vi "loadTestsFromTestCases.vi"(7 "testSuiteStatusChangedRef":refnum<user-event>, 8 "error in (no error)":errorcluster, 10 "Tests":refnum<class>[](array[class]), 11 "TestLoader in":refnum<class "TestLoader.lvclass">) -> (0 "error out":errorcluster, 2 "TestSuite":refnum<class "TestSuite.lvclass">, 3 "TestLoader out":refnum<class "TestLoader.lvclass">)   [LabVIEW 2019, in "TestLoader.lvclass"]
uses:
  TestLoader.lvclass
  TestSuite/TestSuite.lvclass
  TestSuite/suiteStatusChanged--Cluster.ctl
  TestSuite/suiteStatus--enum.ctl
  TestCase/TestCase.lvclass
  <userlib>/_OpenG.lib/array/array.llb/Conditional Auto-Indexing Tunnel (LVObject)__ogtk.vi
  <userlib>/_OpenG.lib/array/array.llb/Conditional Auto-Indexing Tunnel (Variant)__ogtk.vi
  <userlib>/_OpenG.lib/array/array.llb/Filter 1D Array (String)__ogtk.vi
  <userlib>/_OpenG.lib/array/array.llb/Remove Duplicates from 1D Array (I32)__ogtk.vi
  <userlib>/_OpenG.lib/array/array.llb/Delete Elements from 1D Array (LVObject)__ogtk.vi
  Libraries/VITesterUtilities.lvlib
panel:
  # "JKI VI Tester for LabVIEW\nhttp://jkisoft.com/vi-tester\nCopyright (C) 2007-2009, JKI <info@jkisoft.com>\nALL RIGHTS RESERVED"
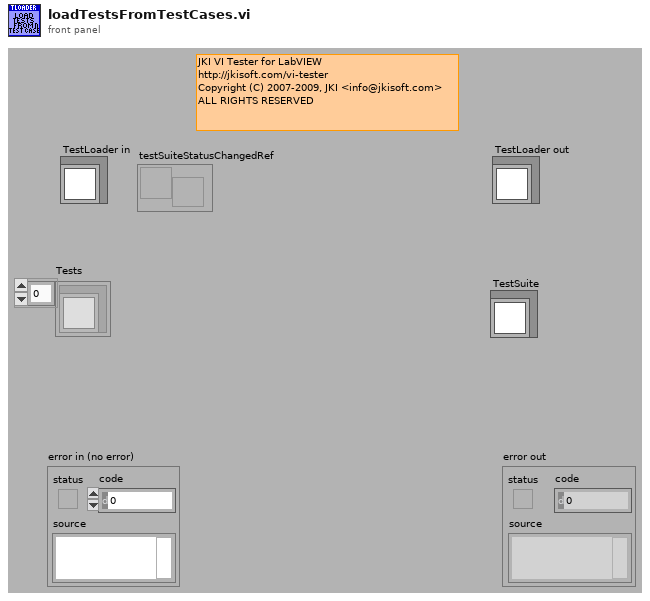
[diagram p1: front panel]
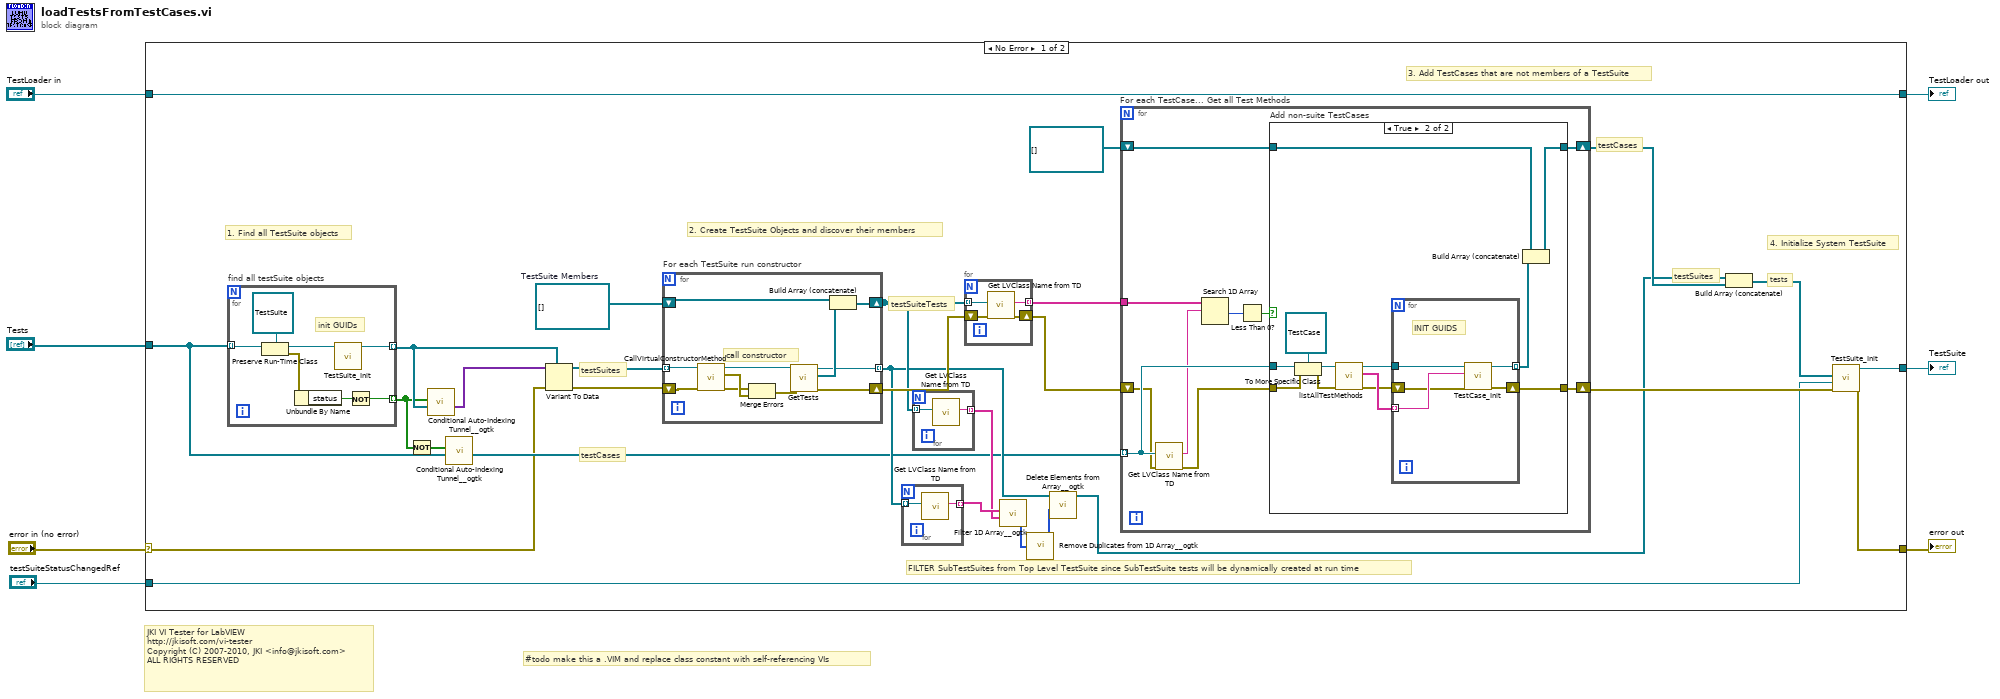
[diagram p0: block diagram]
diagram:
  # "#todo make this a .VIM and replace class constant with self-referencing VIs"
  # "JKI VI Tester for LabVIEW\nhttp://jkisoft.com/vi-tester\nCopyright (C) 2007-2010, JKI <info@jkisoft.com>\nALL RIGHTS RESERVED"
  n1 = case shown="No Error" "error in (no error)" {
    selector: "error in (no error)" -> [w9 w92]
    tunnel: [w32 w92] -> w6
    tunnel: [w35 w91] -> w4
    tunnel: "TestLoader in" -> [w35 w91]
    tunnel: "Tests" -> [w26 _]
    tunnel: [w33 _] -> w2
    tunnel: "testSuiteStatusChangedRef" -> [w18 _]
    frame No Error {
      w24 = refnum<class>[] []  # TestSuite Members
      # "FILTER SubTestSuites from Top Level TestSuite since SubTestSuite tests will be dynamically created at run time"
      # "3. Add TestCases that are not members of a TestSuite"
      # "2. Create TestSuite Objects and discover their members"
      # "1. Find all TestSuite objects"
      # "4. Initialize System TestSuite"
      # "tests"
      # "testCases"
      # "testSuites"
      # "testSuiteTests"
      # "testCases"
      # "testSuites"
      n2 = for "find all testSuite objects" {
        tunnel: w26 -> [w61] mode=indexing
        tunnel: [w55] -> w29 mode=indexing
        tunnel: [w57] -> w28 mode=indexing
        # "init GUIDs"
        n3 = Preserve Run-Time Class(object in=w61, 2:refnum<class "TestSuite.lvclass"> refnum ("reference in")) -> (object out=w56:refnum<class "TestSuite.lvclass">, error out=w59:errorcluster)  [unwired: 1 in]
        n4 = Unbundle By Name(w59) -> ("status"=w58:bool)
        n5 = call "TestSuite_Init.vi"("TestSuite in"=w56) -> ("TestSuite out"=w55:refnum<class "TestSuite.lvclass">)  [unwired: 9 in, 1 out]
        n6 = Not(x=w58) -> (.not. x?=w57:bool)
      }
      n7 = Not(x=w28) -> (.not. x?=w27:bool[])
      n8 = call-poly <userlib>:"Conditional Auto-Indexing Tunnel__ogtk.vi"("Array in"=w29, "Elements to keep"=w28) -> ("Filtered Array out"=w30:variant[])  [unwired: 5 in]
      n9 = call-poly <userlib>:"Conditional Auto-Indexing Tunnel__ogtk.vi"("Array in"=w26, "Elements to keep"=w27) -> ("Filtered Array out"=w10:refnum<class>[])  [unwired: 5 in]
      n10 = Variant To Data(error in=w9, type=w29, Variant=w30) -> (data=w17:refnum<class "TestSuite.lvclass">[], error out=w25:errorcluster)
      n11 = for "For each TestSuite run constructor" {
        tunnel: w17 -> [w49] mode=indexing
        shift-right: [w54] -> w21
        shift-left: w25 -> [w47]
        shift-right: [w51] -> w16
        shift-left: w24 -> [w53]
        tunnel: [w50] -> w13 mode=indexing
        # "call constructor"
        n12 = call "CallVirtualConstructorMethod.vi"("error in"=w47, "TestSuite in"=w49) -> ("error out"=w45:errorcluster, "Constructor Error"=w46:errorcluster, "TestSuite out"=w48:refnum<class "TestSuite.lvclass">)  [unwired: 7 in]
        n13 = Merge Errors(w46, w45) -> (w44:errorcluster)
        n14 = call-dynamic "GetTests.vi"("error in (no error)"=w44, "TestSuite in"=w48) -> ("error out"=w54:errorcluster, "tests"=w52:refnum<class>[], "TestSuite in"=w50:refnum<class "TestSuite.lvclass">)  [unwired: 7 in]
        n15 = Build Array (concatenate)(w53, w52) -> (w51:refnum<class>[])
      }
      n16 = for {
        tunnel: w13 -> [w39] mode=indexing
        tunnel: [w38] -> w15 mode=indexing
        n17 = call "Get LVClass Name from TD.vi"("Variant"=w39) -> ("LVClass Name"=w38:string)  [unwired: 9 in, 1 out]
      }
      n18 = for {
        tunnel: w16 -> [w37] mode=indexing
        tunnel: [w36] -> w14 mode=indexing
        n19 = call "Get LVClass Name from TD.vi"("Variant"=w37) -> ("LVClass Name"=w36:string)  [unwired: 9 in, 1 out]
      }
      n20 = for {
        tunnel: w16 -> [w43] mode=indexing
        shift-right: [w41] -> w20
        shift-left: w21 -> [w42]
        tunnel: [w40] -> w19 mode=indexing
        n21 = call "Get LVClass Name from TD.vi"("error in"=w42, "Variant"=w43) -> ("error out"=w41:errorcluster, "LVClass Name"=w40:string)  [unwired: 8 in]
      }
      n22 = call-poly <userlib>:"Filter 1D Array__ogtk.vi"("items to filter"=w14, "array"=w15) -> ("filtered item indices"=w12:i32[])  [unwired: 4 in, 1 out]
      n23 = call-poly <userlib>:"Remove Duplicates from 1D Array__ogtk.vi"("Input Array"=w12) -> ("Output Array"=w11:i32[])  [unwired: 1 out]
      n24 = call-poly <userlib>:"Delete Elements from Array__ogtk.vi"("indices"=w11, "array"=w13) -> ("array w/ subset deleted"=w8:refnum<class>[])  [unwired: 8 in, 1 out]
      n25 = for "For each TestCase... Get all Test Methods" {
        shift-right: [w71] -> w34
        shift-left: w20 -> [w65]
        shift-right: [w69] -> w23
        shift-left: refnum<class "TestCase.lvclass">[] [] -> [w70]
        tunnel: w10 -> [w66] mode=indexing
        tunnel: w19 -> [w62]
        n26 = call "Get LVClass Name from TD.vi"("error in"=w65, "Variant"=w66) -> ("error out"=w64:errorcluster, "LVClass Name"=w63:string)  [unwired: 8 in]
        n27 = Search 1D Array(1D array=w62, element=w63) -> (index of element=w68:i32)  [unwired: 1 in]
        n28 = Less Than 0?(x=w68) -> (x < 0?=w67:bool)
        n29 = case "Add non-suite TestCases" shown="True" w67 {
          tunnel: [w72 w85] -> w71
          tunnel: w70 -> [w73 w83]
          tunnel: [w73 w82] -> w69
          tunnel: w66 -> [_ w80]
          tunnel: w64 -> [w72 w79]
          frame False {
            # "do not add testCases if testCase is a member of a testSuite"
          }
          frame True {
            n30 = To More Specific Class(target class=refnum<class "TestCase.lvclass"> refnum ("TestCase out"), reference=w80, error in=w79) -> (specific class reference=w78:refnum<class "TestCase.lvclass">, error out=w75:errorcluster)
            n31 = call-dynamic "listAllTestMethods.vi"("error in (no error)"=w75, "TestCase in"=w78) -> ("error out"=w74:errorcluster, "test methods"=w77:string[], "TestCase out"=w76:refnum<class "TestCase.lvclass">)  [unwired: 7 in]
            n32 = for {
              tunnel: w76 -> [w86]
              tunnel: w77 -> [w90] mode=indexing
              shift-right: [w88] -> w85
              shift-left: w74 -> [w87]
              tunnel: [w89] -> w84 mode=indexing
              # "INIT GUIDS"
              n33 = call "TestCase_Init.vi"("error in (no error)"=w87, "methodName (\"runTest\")"=w90, "TestCase in"=w86) -> ("error out"=w88:errorcluster, "TestCase out"=w89:refnum<class "TestCase.lvclass">)  [unwired: 7 in]
            }
            n34 = Build Array (concatenate)(w83, w84) -> (w82:refnum<class "TestCase.lvclass">[])
          }
        }
      }
      n35 = Build Array (concatenate)(w8, w23) -> (w22:refnum<class>[])
      n36 = call "TestSuite_Init.vi"("error in (no error)"=w34, "testSuiteStatusChanged EventRef"=w18, "tests (none)"=w22) -> ("error out"=w32:errorcluster, "TestSuite out"=w33:refnum<class "TestSuite.lvclass">)  [unwired: 7 in]
    }
    frame Error {
    }
  }
  "error out" <- w6
  "TestLoader out" <- w4
  "TestSuite" <- w2
